vi "PhotonUtils_GetYawToPose.vi"(10 "TargetPose":T2={"TRANSLATION"={"X"=0.0, "Y"=0.0}, "ROTATION"={"VALUE"=0.0, "COS"=1.0, "SIN"=0.0}} {"ROTATION"."SIN" format="%13.4f"; "ROTATION"."COS" format="%13.4f"; "ROTATION"."VALUE" format="%13.4f"; "TRANSLATION"."Y" format="%14.3f"; "TRANSLATION"."X" format="%14.3f"}, 11 "RobotPose":T2={"TRANSLATION"={"X"=0.0, "Y"=0.0}, "ROTATION"={"VALUE"=0.0, "COS"=1.0, "SIN"=0.0}} {"ROTATION"."SIN" format="%13.4f"; "ROTATION"."COS" format="%13.4f"; "ROTATION"."VALUE" format="%13.4f"; "TRANSLATION"."Y" format="%14.3f"; "TRANSLATION"."X" format="%14.3f"}) -> (3 "YawToPose":T1={"VALUE"=0.0, "COS"=1.0, "SIN"=0.0} {"SIN" format="%13.4f"; "COS" format="%13.4f"; "VALUE" format="%13.4f"})   [LabVIEW 2019, in "PhotonVisionLib.lvlib"]
doc: "Returns the yaw between your robot and a target.\n\nInputs:\n - RobotPose -- Pose2d of the robot.\n - TargetPose -- Pose2d of the target\n\nOutputs\n - YawToPose -- Yaw to the target"
uses:
  <vilib>/Rock Robotics/WPI/ThirdParty/JAS_Junk/TrajLib/TypeDef/POSE2D.ctl
  <vilib>/Rock Robotics/WPI/ThirdParty/JAS_Junk/TrajLib/TypeDef/TRANSLATION2D.ctl
  <vilib>/Rock Robotics/WPI/ThirdParty/JAS_Junk/TrajLib/TypeDef/ROTATION2D.ctl
  <vilib>/Rock Robotics/WPI/ThirdParty/JAS_Junk/TrajLib/Util_CalcDist.vi
  PhotonVisionLib.lvlib
  <vilib>/Rock Robotics/WPI/ThirdParty/JAS_Junk/TrajLib/Trajectory_Library.lvlib
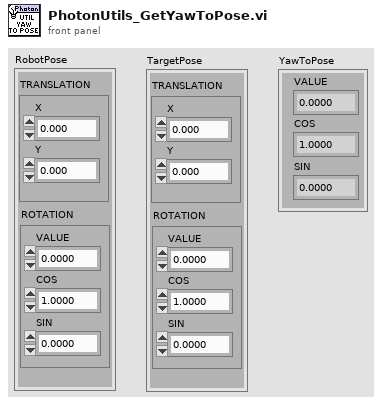
[diagram p1: front panel]
types:
  T1 = typedef "Trajectory_Library.lvlib/ROTATION2D.ctl" = cluster{"VALUE":dbl, "COS":dbl, "SIN":dbl}
  T2 = typedef "Trajectory_Library.lvlib/POSE2D.ctl" = cluster{"TRANSLATION":T3, "ROTATION":T1}
  T3 = typedef "Trajectory_Library.lvlib/TRANSLATION2D.ctl" = cluster{"X":dbl, "Y":dbl}
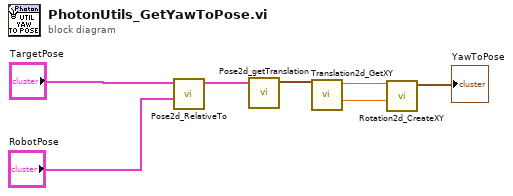
[diagram p0: block diagram]
diagram:
  n1 = call <vilib>:"Pose2d_RelativeTo.vi"("other POSE"="RobotPose", "in POSE"="TargetPose") -> ("out POSE"=w5:T2)  [unwired: 9 in]
  n2 = call <vilib>:"Pose2d_getTranslation.vi"("in POSE"=w5) -> ("outTRANSLATION"=w4:T3)  [unwired: 10 in]
  n3 = call <vilib>:"Translation2d_GetXY.vi"("In Translation"=w4) -> ("Y"=w2:dbl, "X"=w3:dbl)  [unwired: 9 in]
  n4 = call <vilib>:"Rotation2d_CreateXY.vi"("Y or sine"=w2, "X or  cosine"=w3) -> ("ROTATION"=→"YawToPose":T1)  [unwired: 9 in]
